vi "PC main.vi"() -> ()   [LabVIEW 2019]
panel:
  out "u data":dbl[](array[numeric])
  out "j data":dbl[](array[numeric])
  out "dx data":dbl[](array[numeric])
  out "x data":dbl[](array[numeric])
  out "Wait for  CL ready":bool
  in  "u data path":path=path "C:/RT_MLC/u_data.txt"
  in  "j data path":path=path "C:/RT_MLC/j_data.txt"
  in  "dx data path":path=path "C:/RT_MLC/dx_data.txt"
  in  "x data path":path=path "C:/RT_MLC/x_data.txt"
  out "Wait for  PD":bool
  out "Wait for Ind":bool
  in  "Cost path":path=path "C:/RT_MLC/cost.txt"
  in  "Cost Ready path":path=path "C:/RT_MLC/costReady.txt"
  in  "CL path":path=path "C:/RT_MLC/controlLaw.txt"
  in  "CL Ready path":path=path "C:/RT_MLC/controlLawReady.txt"
  out "Run Time":dbl
  in  "stop":bool
  in  "Individual Time[s]":dbl=0.5
  in  "PD Time[s]":dbl=0.6
  out "J":dbl
  out "Control Law":string
  out "PD":bool
  out "Run flag":bool
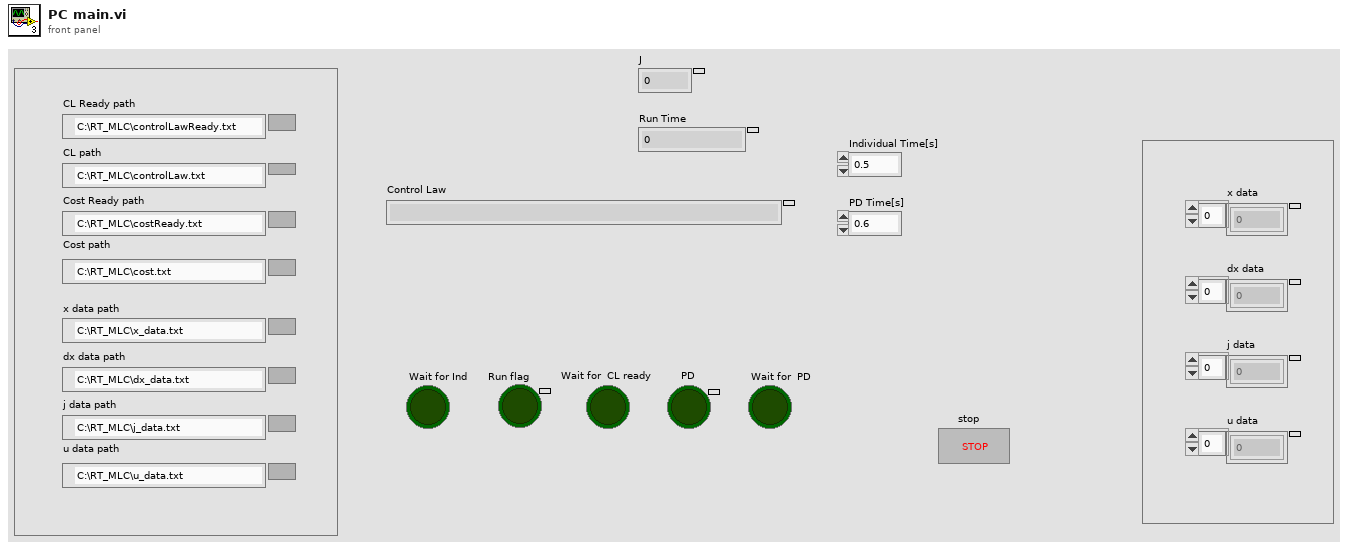
[diagram p1: front panel]
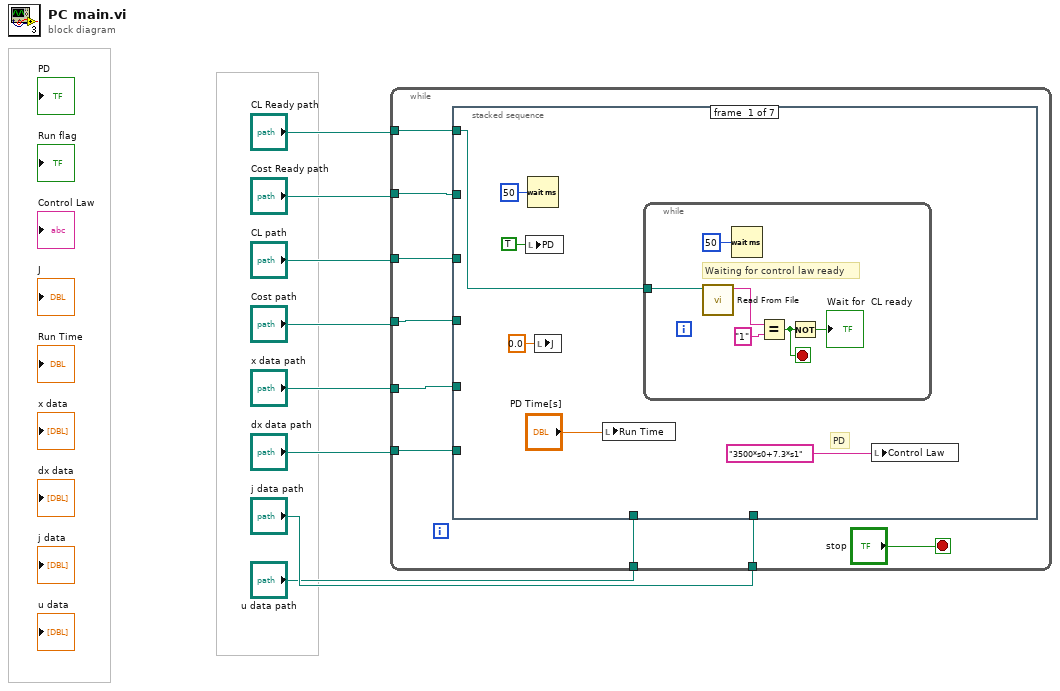
[diagram p0: block diagram]
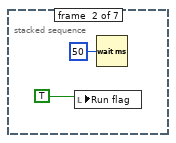
[diagram p2: hidden frame]
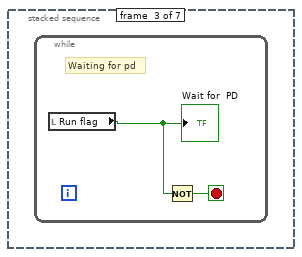
[diagram p3: hidden frame]
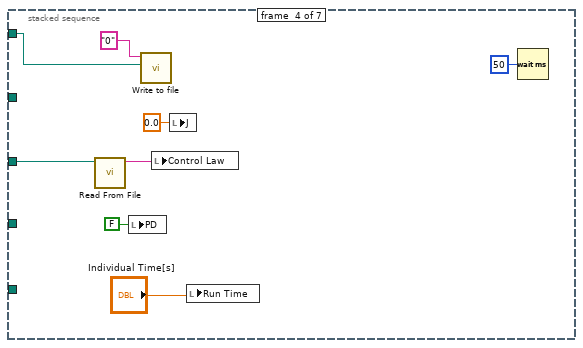
[diagram p4: hidden frame]
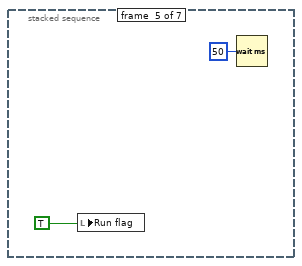
[diagram p5: hidden frame]
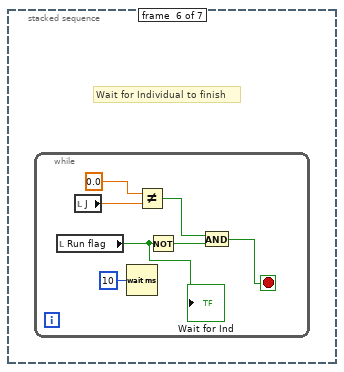
[diagram p6: hidden frame]
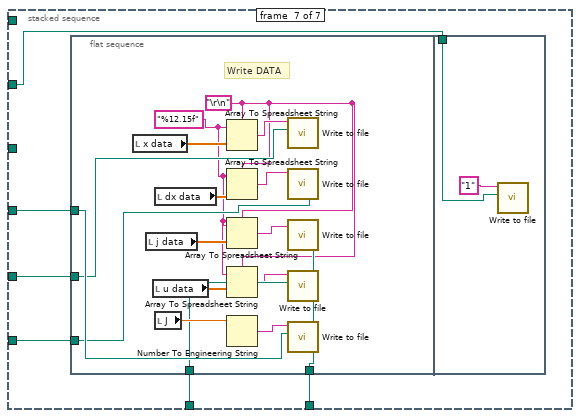
[diagram p7: hidden frame]
diagram:
  n1 = while {
    tunnel: "CL path" -> [w17]
    tunnel: "Cost path" -> [w16]
    tunnel: "CL Ready path" -> [w15]
    tunnel: "Cost Ready path" -> [w14]
    tunnel: "x data path" -> [w12]
    tunnel: "dx data path" -> [w11]
    tunnel: "j data path" -> [w10]
    tunnel: "u data path" -> [w9]
    stop <- "stop" stop-if-true
    n2 = stacked-sequence {
      tunnel: w15 -> [w18 _ _ w37 _ _ _]
      tunnel: w17 -> [_ _ _ w36 _ _ _]
      tunnel: w16 -> [_ _ _ _ _ _ w56]
      tunnel: w14 -> [_ _ _ _ _ _ w55]
      tunnel: w12 -> [_ _ _ _ _ _ w54]
      tunnel: w11 -> [_ _ _ _ _ _ w53]
      tunnel: w10 -> [_ _ _ _ _ _ w52]
      tunnel: w9 -> [_ _ _ _ _ _ w51]
      frame #0 {
        # "PD"
        n3 = local write "PD"(TRUE ("PD")) -> ()
        n4 = Wait (ms)(milliseconds to wait=u32 50) -> ()  [unwired: 1 out]
        n5 = local write "J"(0.0 ("J")) -> ()
        n6 = local write "Run Time"("PD Time[s]") -> ()
        n7 = while {
          tunnel: w18 -> [w24]
          stop <- w25 stop-if-true
          # "Waiting for control law ready"
          n8 = call "Read From File.vi"("file path (use dialog)"=w24) -> ("String"=w27:string)  [unwired: 10 in]
          n9 = Wait (ms)(milliseconds to wait=u32 50) -> ()  [unwired: 1 out]
          n10 = Equal?(x=w27, y="1") -> (x = y?=w25:bool)
          n11 = Not(x=w25) -> (.not. x?=→"Wait for  CL ready":bool)
        }
        n12 = local write "Control Law"("3500*s0+7.3*s1") -> ()
      }
      frame #1 {
        n13 = local write "Run flag"(TRUE ("run_flag")) -> ()
        n14 = Wait (ms)(milliseconds to wait=u32 50) -> ()  [unwired: 1 out]
      }
      frame #2 {
        n15 = while {
          stop <- w32 stop-if-true
          # "Waiting for pd"
          n16 = local read "Run flag"() -> (w33:bool)
          "Wait for  PD" <- w33
          n17 = Not(x=w33) -> (.not. x?=w32:bool)
        }
      }
      frame #3 {
        n18 = call "Read From File.vi"("file path (use dialog)"=w36) -> ("String"=w39:string)  [unwired: 10 in]
        n19 = local write "PD"(FALSE ("PD")) -> ()
        n20 = call "Write to file.vi"("file path (use dialog)"=w37, "String"="0" ("text")) -> ()  [unwired: 10 in]
        n21 = local write "Control Law"(w39) -> ()
        n22 = local write "J"(0.0 ("J")) -> ()
        n23 = local write "Run Time"("Individual Time[s]") -> ()
        n24 = Wait (ms)(milliseconds to wait=u32 50) -> ()  [unwired: 1 out]
      }
      frame #4 {
        n25 = local write "Run flag"(TRUE ("run_flag")) -> ()
        n26 = Wait (ms)(milliseconds to wait=u32 50) -> ()  [unwired: 1 out]
      }
      frame #5 {
        # "Wait for Individual to finish"
        n27 = while {
          stop <- w45 stop-if-true
          n28 = local read "Run flag"() -> (w44:bool)
          "Wait for Ind" <- w44
          n29 = local read "J"() -> (w49:dbl)
          n30 = Wait (ms)(milliseconds to wait=u32 10) -> ()  [unwired: 1 out]
          n31 = Not Equal?(x=0.0, y=w49) -> (x != y?=w46:bool)
          n32 = Not(x=w44) -> (.not. x?=w47:bool)
          n33 = And(x=w46, y=w47) -> (x .and. y?=w45:bool)
        }
      }
      frame #6 {
        n34 = flat-sequence {
          tunnel: w56 -> [w71]
          tunnel: w54 -> [w70]
          tunnel: w53 -> [w69]
          tunnel: w52 -> [w68]
          tunnel: w51 -> [w67]
          tunnel: w55 -> [w74]
          frame #0 {
            w57 = "\r\n"
            w58 = "%12.15f" ("format string")
            # "Write DATA"
            n35 = local read "x data"() -> (w66:dbl[])
            n36 = local read "j data"() -> (w64:dbl[])
            n37 = local read "u data"() -> (w65:dbl[])
            n38 = local read "dx data"() -> (w63:dbl[])
            n39 = local read "J"() -> (w72:dbl)
            n40 = Array To Spreadsheet String(delimiter (Tab)=w57, array=w66, 3:w58) -> (spreadsheet string=w59:string)
            n41 = Array To Spreadsheet String(delimiter (Tab)=w57, array=w63, 3:w58) -> (spreadsheet string=w60:string)
            n42 = Array To Spreadsheet String(delimiter (Tab)=w57, array=w64, 3:w58) -> (spreadsheet string=w61:string)
            n43 = Array To Spreadsheet String(delimiter (Tab)=w57, array=w65, 3:w58) -> (spreadsheet string=w62:string)
            n44 = Number To Engineering String(4:w72) -> (0:w73:string)  [unwired: 3 in]
            n45 = call "Write to file.vi"("file path (use dialog)"=w70, "String"=w59) -> ()  [unwired: 10 in]
            n46 = call "Write to file.vi"("file path (use dialog)"=w69, "String"=w60) -> ()  [unwired: 10 in]
            n47 = call "Write to file.vi"("file path (use dialog)"=w68, "String"=w61) -> ()  [unwired: 10 in]
            n48 = call "Write to file.vi"("file path (use dialog)"=w67, "String"=w62) -> ()  [unwired: 10 in]
            n49 = call "Write to file.vi"("file path (use dialog)"=w71, "String"=w73) -> ()  [unwired: 10 in]
          }
          frame #1 {
            n50 = call "Write to file.vi"("file path (use dialog)"=w74, "String"="1" ("text")) -> ()  [unwired: 10 in]
          }
        }
      }
    }
  }
